vi "Construct.vi"(8 "error in (no error)":errorcluster, 9 "Request URI":string, 10 "Success?":bool=TRUE, 11 "ErrorOrSuccess in":refnum<class "ErrorOrSuccess.lvclass">) -> (0 "error out":errorcluster, 3 "ErrorOrSuccess out":refnum<class "ErrorOrSuccess.lvclass">)   [LabVIEW 2020, in "wamplv.lvlib" / "ErrorOrSuccess.lvclass"]
uses:
  ErrorOrSuccess.lvclass
  ErrorOrSuccess.lvclass/ErrorOrSuccess.ctl
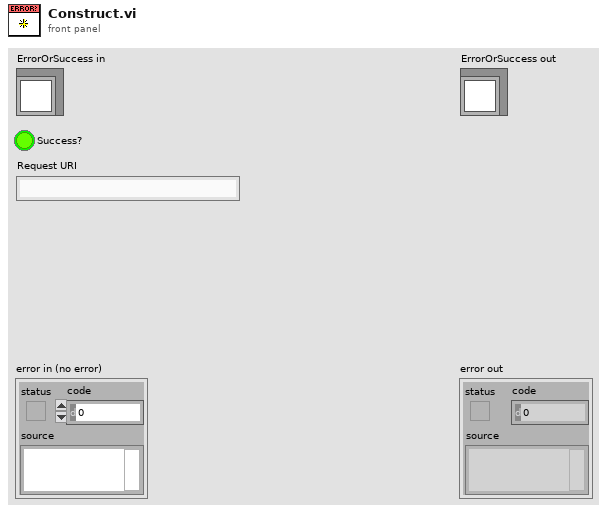
[diagram p1: front panel]
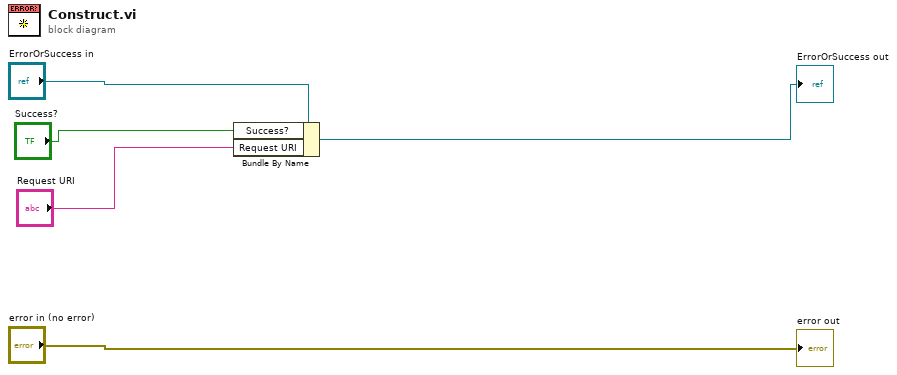
[diagram p0: block diagram]
diagram:
  n1 = Bundle By Name(cluster="ErrorOrSuccess in", "Success?"="Success?", "Request URI"="Request URI") -> (→"ErrorOrSuccess out":refnum<class "ErrorOrSuccess.lvclass">)
  "error out" <- "error in (no error)"
